vi "magnet ps selection.vi"() -> (0 "Magnet PS":u16(ring)=1 items=["Resistive Magnet", "SCM2", "SCM1", "Generic SC power supply"])   [LabVIEW 2019]
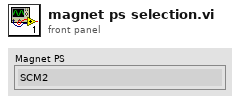
[diagram p1: front panel]
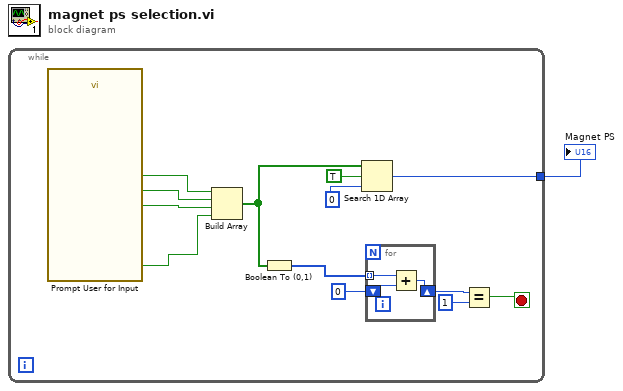
[diagram p0: block diagram]
diagram:
  n1 = while {
    tunnel: [w2] -> w1
    stop <- w10 stop-if-true
    n2 = call "Prompt User for Input"() -> ("Generic SC power supply"=w11:bool, "SCM1 magnet"=w12:bool, "SCM2 magnet"=w13:bool, "Resistive magnet"=w14:bool)  [unwired: 14 in, 2 out]
    n3 = Build Array(w14, w13, w12, w11) -> (w5:bool[])
    n4 = Boolean To (0,1)(Boolean=w5) -> (0, 1=w9:i16[])
    n5 = Search 1D Array(1D array=w5, element=TRUE, start index (0)=0 ("index of element")) -> (index of element=w2:i32)
    n6 = for {
      tunnel: w9 -> [w17] mode=indexing
      shift-right: [w16] -> w7
      shift-left: i16 0 -> [w15]
      n7 = Add(x=w17, y=w15) -> (x+y=w16:i16)
    }
    n8 = Equal?(x=w7, y=i16 1) -> (x = y?=w10:bool)
  }
  "Magnet PS" <- w1
